vi "Auto - Values into Cluster (SubVI).vi"(6 "Auto Array":dbl[][](array[numeric]), 7 "Was Disabled":bool, 11 "Auton State":i32) -> (1 "Auton Input Cluster With Data":T1, 3 "Auton State Out":i32)   [LabVIEW 2020]
uses:
  TypeDefs/Auton Cluster Typedef.ctl
panel:
  in  "Auton Input Cluster in":T1
  # "Controls"
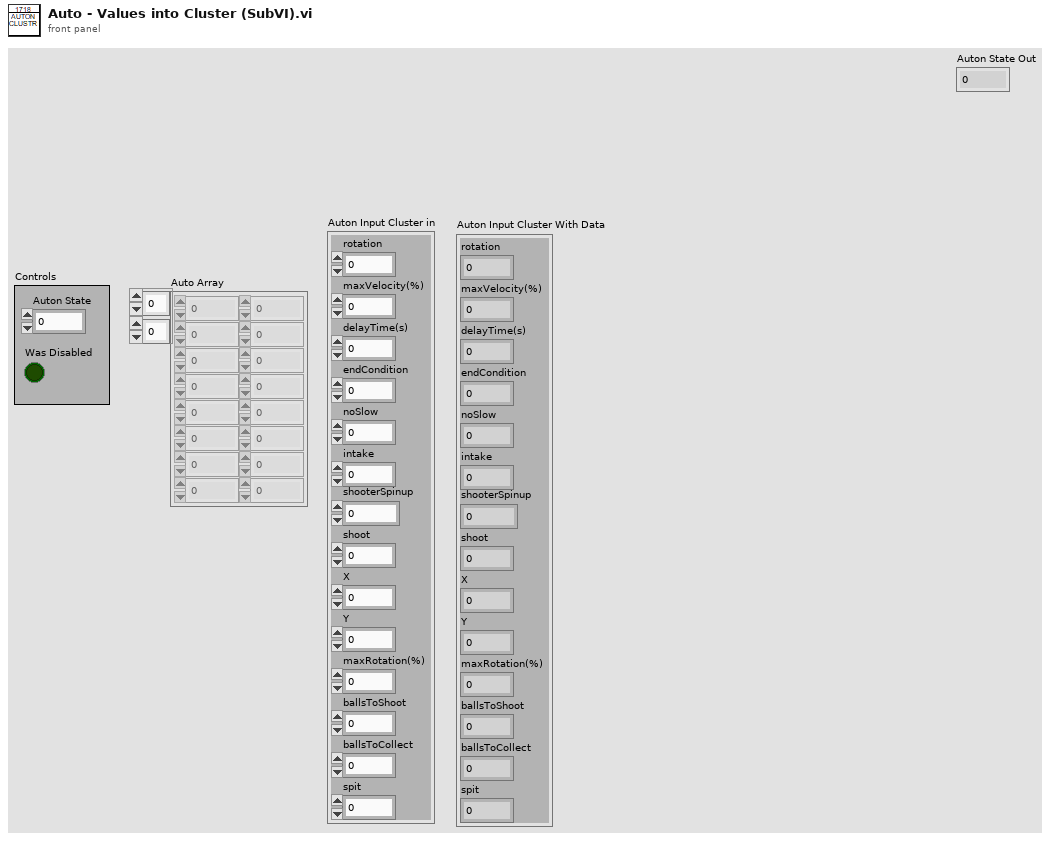
[diagram p1: front panel]
types:
  T1 = typedef "Auton Cluster Typedef.ctl" = cluster{"rotation":dbl, "maxVelocity(%)":dbl, "delayTime(s)":dbl, "endCondition":dbl, "noSlow":dbl, "intake":dbl, "shooterSpinup":dbl, "shoot":dbl, "X":dbl, "Y":dbl, "maxRotation(%)":dbl, "ballsToShoot":dbl, "ballsToCollect":dbl, "spit":dbl}
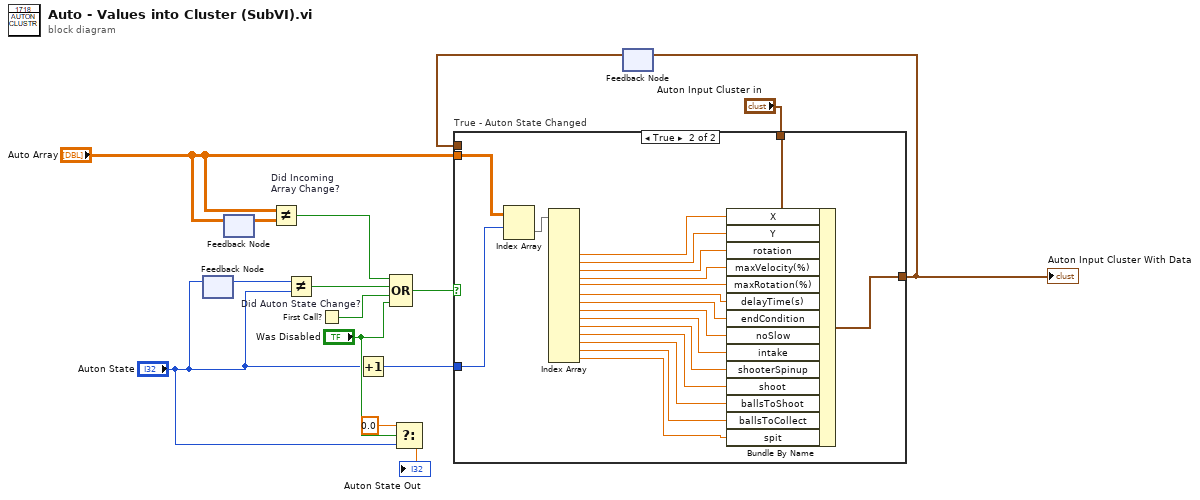
[diagram p0: block diagram]
diagram:
  n1 = feedback-in #1("Auton State") -> ()
  n2 = feedback #1() -> (w6:i32)  [unwired: 1 in]
  n3 = feedback #2() -> (w12:dbl[][])  [unwired: 1 in]
  n4 = feedback-in #2("Auto Array") -> ()
  n5 = Not Equal? "Did Incoming\nArray Change?"(x="Auto Array", y=w12) -> (x != y?=w8:bool)
  n6 = Not Equal? "Did Auton State Change?"(x=w6, y="Auton State") -> (x != y?=w11:bool)
  n7 = First Call?() -> (First Call?: T/F=w10:bool)
  n8 = Increment(x="Auton State") -> (x+1=w5:i32)
  n9 = Compound Arithmetic op=OR(w8, w11, w10, "Was Disabled") -> (w9:bool)
  n10 = Select(t=0.0, s="Was Disabled", f="Auton State") -> (s? t:f=→"Auton State Out":dbl)
  n11 = feedback #3() -> (w13:T1)  [unwired: 1 in]
  n12 = case "True - Auton State Changed" shown="True" w9 {
    tunnel: [w16 w35] -> w14
    tunnel: "Auton Input Cluster in" -> [_ w34]
    tunnel: w5 -> [_ w33]
    tunnel: w13 -> [w16 _]
    tunnel: "Auto Array" -> [_ w32]
    frame False {
    }
    frame True {
      n13 = Index Array(array=w32, index (row)=w33) -> (element=w31:dbl[])  [unwired: 1 in]
      n14 = Index Array(array=w31) -> (element #4=w30:dbl, element #5=w29:dbl, element #6=w28:dbl, element #7=w27:dbl, element #8=w26:dbl, element #9=w25:dbl, element #10=w24:dbl, element #11=w23:dbl, element #12=w22:dbl, element #13=w21:dbl, element #14=w20:dbl, element #15=w19:dbl, element #16=w18:dbl, element #17=w17:dbl)  [unwired: 17 in, 3 out]
      n15 = Bundle By Name(cluster=w34, "X"=w30, "Y"=w29, "rotation"=w28, "maxVelocity(%)"=w27, "maxRotation(%)"=w26, "delayTime(s)"=w25, "endCondition"=w24, "noSlow"=w23, "intake"=w22, "shooterSpinup"=w21, "shoot"=w20, "ballsToShoot"=w19, "ballsToCollect"=w18, "spit"=w17) -> (w35:T1)
    }
  }
  "Auton Input Cluster With Data" <- w14
  n16 = feedback-in #3(w14) -> ()
